vi "Cleanup.vi"(8 "error in (no error)":errorcluster, 11 "Mouse in":refnum<class "Mouse.lvclass">) -> (0 "error out":errorcluster)   [LabVIEW 2020, in "Maze.lvlib" / "Mouse.lvclass"]
doc: "This VI is called when unloading the mouse and is useful when you've initialized resources in the <i>Init.vi</i>. If you created any DVRs, Queues, etc. in <i>Init.vi</i> you should release those resources here.\n\nThis VI is only called in preparation of loading a new mouse class or shutting down the application."
uses:
  Mouse.lvclass
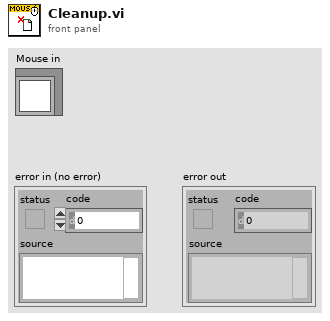
[diagram p1: front panel]
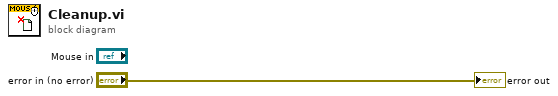
[diagram p0: block diagram]
diagram:
  "error out" <- "error in (no error)"
